vi "Open_Command_Table.vi"() -> (1 "Commands":cluster{string, string[]}[](array[cluster]), 2 "Alias Table":string[][](array[string]))   [LabVIEW 2011]
doc: "This VI opens and parses \"command_table.txt\", which is stored on the local filesystem in the same directory as this VI. It outputs a cluster array, each element containing a command and an array of arguments available for that command (strings). It also outputs an alias table, which is a 2d array of strings. The first row contains the formal commands, and the second row contains the command aliases."
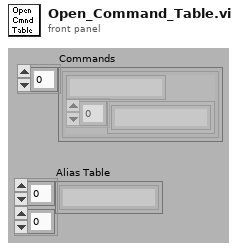
[diagram p1: front panel]
types:
  T1 = cluster{"Start Row":i32, "Start Column":i32, "End Row":i32, "End Column":i32}
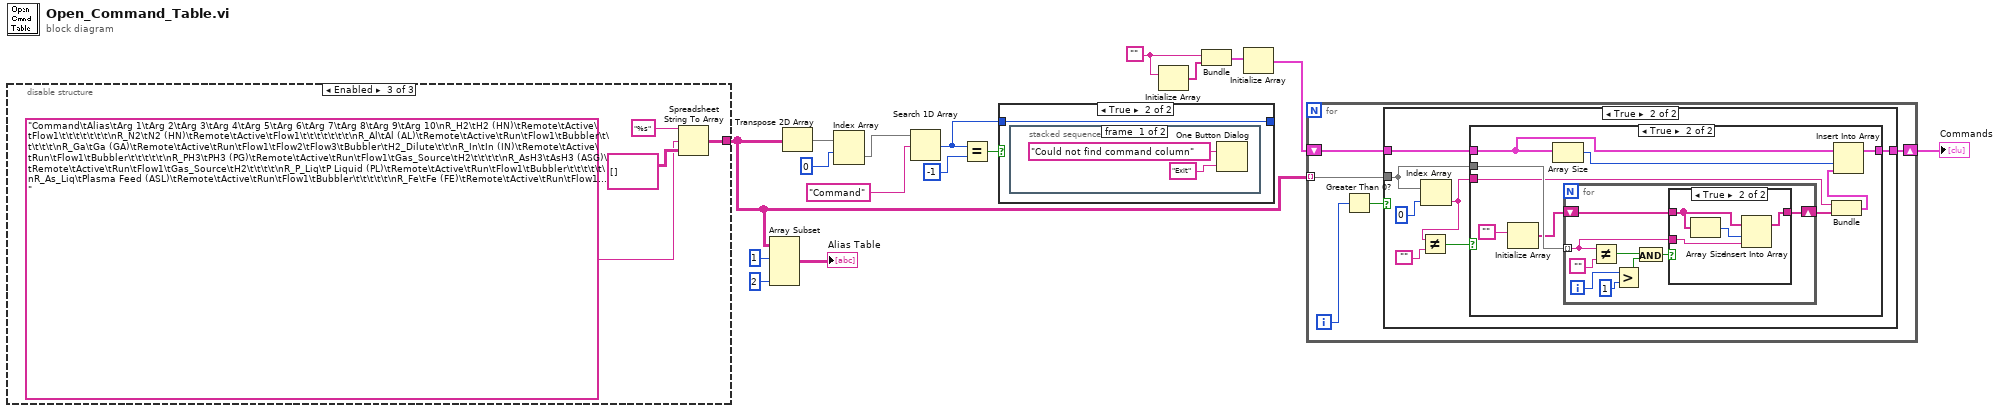
[diagram p0: block diagram]
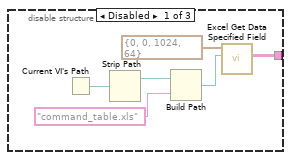
[diagram p2: hidden frame]
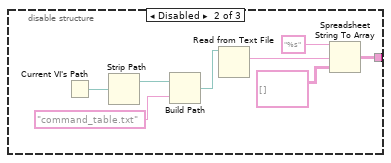
[diagram p3: hidden frame]
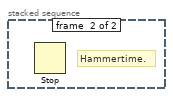
[diagram p8: hidden frame]
diagram:
  w9 = ""
  n1 = disable-structure shown="Enabled" {
    disable-tunnel: [w17 w23 w32] -> w1
    frame Disabled {
      n2 = Current VI's Path() -> (path=w20:path)
      n3 = Strip Path(path=w20) -> (stripped path=w19:path)  [unwired: 1 out]
      n4 = Build Path(base path=w19, name or relative path="command_table.xls") -> (appended path=w18:path)
      n5 = call "Excel Get Data Specified Field.vi"("file path"=w18, "Start and End"=T1 {"Start Row"=0, "Start Column"=0, "End Row"=1024, "End Column"=64}) -> ("data"=w17:string[][])  [unwired: 2 in, 3 out]
    }
    frame Disabled {
      n6 = Current VI's Path() -> (path=w27:path)
      n7 = Strip Path(path=w27) -> (stripped path=w28:path)  [unwired: 1 out]
      n8 = Build Path(base path=w28, name or relative path="command_table.txt") -> (appended path=w25:path)
      n9 = Read from Text File(file (use dialog)=w25) -> (text=w24:string)  [unwired: 1 in, 5 out]
      n10 = Spreadsheet String To Array(format string="%s", spreadsheet string=w24, array type (2D Dbl)=string[][] [] ("data")) -> (array=w23:string[][])  [unwired: 1 out]
    }
    frame Enabled {
      n11 = Spreadsheet String To Array(format string="%s", spreadsheet string="Command\tAlias\tArg 1\tArg 2\tArg 3\tArg 4\tArg 5\tArg 6\tArg 7\tArg 8\tArg 9\tArg 10\nR_H2\tH2 (HN)\tRemote\tActive\tFlow1\t\t\t\t\t\t\t\nR_N2\tN2 (HN)\tRemote\tActive\tFlow1\t\t\t\t\t\t\t\nR_Al\tAl (AL)\tRemote\tActive\tRun\tFlow1\tBubbler\t\t\t\t\t\nR_Ga\tGa (GA)\tRemote\tActive\tRun\tFlow1\tFlow2\tFlow3\tBubbler\tH2_Dilute\t\t\nR_In\tIn (IN)\tRemote\tActive\tRun\tFlow1\tBubbler\t\t\t\t\t\nR_PH3\tPH3 (PG)\tRemote\tActive\tRun\tFlow1\tGas_Source\tH2\t\t\t\t\nR_AsH3\tAsH3 (ASG)\tRemote\tActive\tRun\tFlow1\tGas_Source\tH2\t\t\t\t\nR_P_Liq\tP Liquid (PL)\tRemote\tActive\tRun\tFlow1\tBubbler\t\t\t\t\t\nR_As_Liq\tPlasma Feed (ASL)\tRemote\tActive\tRun\tFlow1\tBubbler\t\t\t\t\t\nR_Fe\tFe (FE)\tRemote\tActive\tRun\tFlow1\tFlow2\tFlow3\tBubbler\tH2_Dilute\t\t\nR_P_Dop\tp Dopant (PDOP)\tRemote\tActive\tRun\tFlow1\tFlow2\tFlow3\tFlow4\tBubbler\tH2_Dilute\tGas_Source\nR_N_Dop\tn Dopant (NDOP)\tRemote\tActive\tRun\tFlow1\tFlow2\tFlow3\tFlow4\tBubbler\tH2_Dilute\tGas_Source\nH_Heater\tHeater\tRemote\tHeater\tSpinner\t\t\t\t\t\t\t\nV_Vacuum\tVacuum\tVac_Exhaust\tAtm_Exhaust\t\t\t\t\t\t\t\t\nT_Set_Temp\tSet Temperature\tTemperature\t\t\t\t\t\t\t\t\t\nW_Wait\tWait\t\t\t\t\t\t\t\t\t\t\nL_Loop\tLoop\t", array type (2D Dbl)=string[][] [] ("data")) -> (array=w32:string[][])  [unwired: 1 out]
    }
  }
  n12 = Array Subset(array=w1, index (row)=1 ("index"), length (col)=2 ("length")) -> (→"Alias Table":string[][])  [unwired: 2 in]
  n13 = Transpose 2D Array(2D array=w1) -> (transposed array=w5:string[][])
  n14 = Index Array(array=w5, index (row)=0) -> (element=w11:string[])  [unwired: 1 in]
  n15 = Search 1D Array(1D array=w11, element="Command") -> (index of element=w12:i32)  [unwired: 1 out]
  n16 = Equal?(x=w12, y=-1) -> (x = y?=w13:bool)
  n17 = case shown="True" w13 {
    tunnel: [w35 w36] -> _
    tunnel: w12 -> [w35 w36]
    frame False {
    }
    frame True {
      n18 = stacked-sequence {
        frame #0 {
          n19 = One Button Dialog(message="Could not find command column", button name ("OK")="Exit") -> ()  [unwired: 1 out]
        }
        frame #1 {
          # "Hammertime."
          n20 = Stop() -> ()  [unwired: 1 out]
        }
      }
    }
  }
  n21 = Initialize Array(w9) -> (w10:string[])  [unwired: 1 out]
  n22 = Bundle(w9, w10) -> (w8:cluster{string, string[]})  [unwired: 1 out]
  n23 = Initialize Array(w8) -> (w7:cluster{string, string[]}[])  [unwired: 1 out]
  n24 = for {
    shift-right: [w42] -> w6
    shift-left: w7 -> [w41]
    tunnel: w1 -> [w40] mode=indexing
    i -> [w39]
    n25 = Greater Than 0?(x=w39) -> (x > 0?=w43:bool)
    n26 = case shown="True" w43 {
      tunnel: w40 -> [_ w47]
      tunnel: [w44 w50] -> w42
      tunnel: w41 -> [w44 w49]
      frame False {
      }
      frame True {
        n27 = Index Array(array=w47, index=0) -> (element=w45:string)
        n28 = Not Equal?(x=w45, y="") -> (x != y?=w46:bool)
        n29 = case shown="True" w46 {
          tunnel: w47 -> [_ w57]
          tunnel: [w52 w59] -> w50
          tunnel: w49 -> [w52 w60]
          tunnel: w45 -> [_ w55]
          frame False {
          }
          frame True {
            n30 = Initialize Array("") -> (w56:string[])  [unwired: 1 out]
            n31 = Array Size(array=w60) -> (size(s)=w61:i32)
            n32 = for {
              tunnel: w57 -> [w67] mode=indexing
              shift-right: [w68] -> w54
              shift-left: w56 -> [w69]
              i -> [w63]
              n33 = Not Equal?(x=w67, y="") -> (x != y?=w65:bool)
              n34 = Greater?(x=w63, y=1) -> (0:w64:bool)
              n35 = And(x=w65, y=w64) -> (x .and. y?=w66:bool)
              n36 = case shown="True" w66 {
                tunnel: w69 -> [w71 w74]
                tunnel: [w71 w72] -> w68
                tunnel: w67 -> [_ w73]
                frame False {
                }
                frame True {
                  n37 = Array Size(array=w74) -> (size(s)=w75:i32)
                  n38 = Insert Into Array(array=w74, index=w75, new element=w73) -> (w72:string[])
                }
              }
            }
            n39 = Bundle(w55, w54) -> (w53:cluster{string, string[]})  [unwired: 1 out]
            n40 = Insert Into Array(array=w60, index=w61, new element=w53) -> (w59:cluster{string, string[]}[])
          }
        }
      }
    }
  }
  "Commands" <- w6
